vi "lunch menu 2 sub vi.vi"() -> (1 "potato":string, 2 "veg":string, 3 "entree":string, 4 "grilled sandy":string)   [LabVIEW 2019]
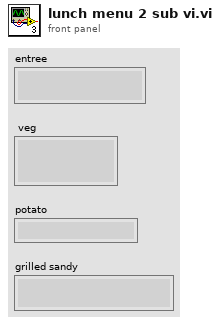
[diagram p1: front panel]
types:
  T1 = cluster{"menu-id":string, "data":cluster{"Lunch":cluster{"GRILLED SANDWICH":string[], "POTATO & RICE ACCOMPANIMENTS":string[], "VEGETABLES":string[], "LUNCH ENTREE":string[]}}}
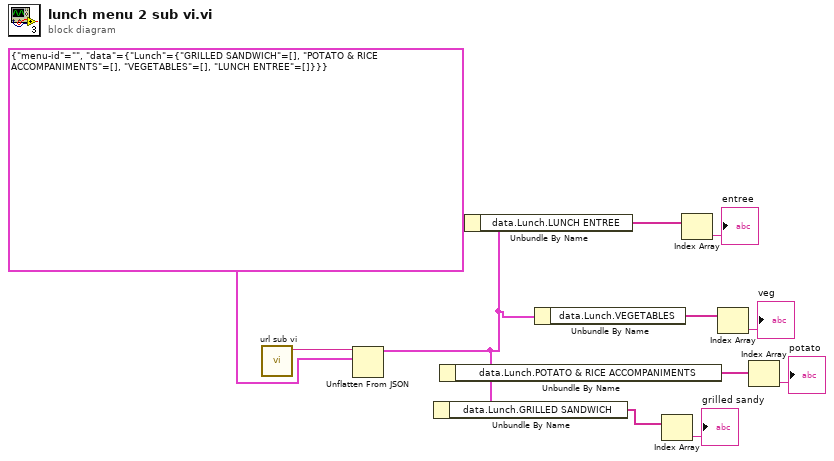
[diagram p0: block diagram]
diagram:
  n1 = call "url sub vi.vi"() -> ("body 2"=w1:string)  [unwired: 11 in]
  n2 = Unflatten From JSON(JSON string=w1, type and defaults=T1 {"menu-id"="", "data"={"Lunch"={"GRILLED SANDWICH"=[], "POTATO & RICE ACCOMPANIMENTS"=[], "VEGETABLES"=[], "LUNCH ENTREE"=[]}}}) -> (value=w3:T1)  [unwired: 5 in, 1 out]
  n3 = Unbundle By Name(w3) -> ("data.Lunch.GRILLED SANDWICH"=w4:string[])
  n4 = Unbundle By Name(w3) -> ("data.Lunch.POTATO & RICE ACCOMPANIMENTS"=w5:string[])
  n5 = Unbundle By Name(w3) -> ("data.Lunch.LUNCH ENTREE"=w7:string[])
  n6 = Unbundle By Name(w3) -> ("data.Lunch.VEGETABLES"=w6:string[])
  n7 = Index Array(array=w4) -> (element=→"grilled sandy":string)  [unwired: 1 in]
  n8 = Index Array(array=w7) -> (element=→"entree":string)  [unwired: 1 in]
  n9 = Index Array(array=w6) -> (element=→"veg":string)  [unwired: 1 in]
  n10 = Index Array(array=w5) -> (element=→"potato":string)  [unwired: 1 in]
